vi "Get RTPath String.vi"(8 "error in (no error)":errorcluster, 11 "Target OS in":string) -> (0 "error out":errorcluster, 1 "RT Folder Path":string, 2 "RT File Path":string, 3 "Target OS out":string)   [LabVIEW 2019, in "TLCD System Tests.lvclass"]
uses:
  TLCD System Tests.lvclass
  TLCD Test Class/TLCD Test Class.lvclass
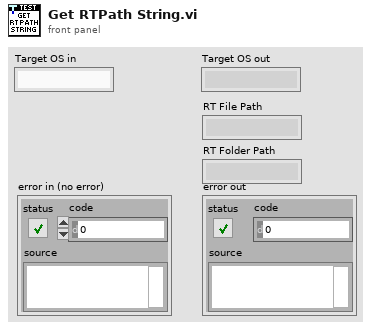
[diagram p1: front panel]
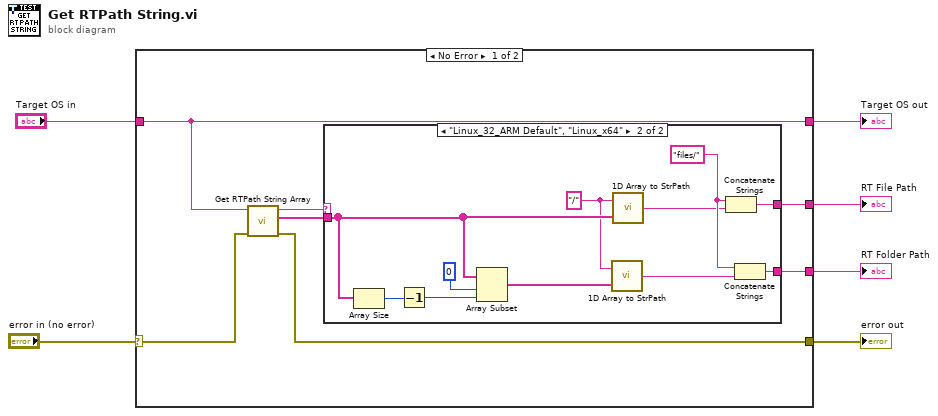
[diagram p0: block diagram]
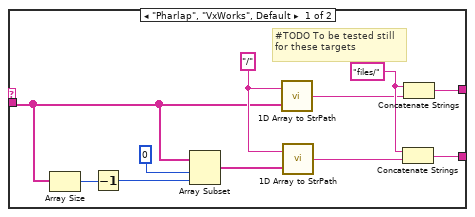
[diagram p2: hidden frame]
diagram:
  n1 = case shown="No Error" "error in (no error)" {
    selector: "error in (no error)" -> [w9 w36]
    tunnel: [w13 _] -> w6
    tunnel: [w12 w36] -> w5
    tunnel: "Target OS in" -> [w8 w37]
    tunnel: [w8 w37] -> w2
    tunnel: [w7 _] -> w1
    frame No Error {
      n2 = call "Get RTPath String Array.vi"("error in (no error)"=w9, "Target OS"=w8) -> ("error out"=w12:errorcluster, "File Path String Array"=w11:string[], "Target OS out"=w10:string)  [unwired: 7 in]
      n3 = case shown="\"Linux_32_ARM Default\", \"Linux_x64\"" w10 {
        tunnel: w11 -> [w16 w31]
        tunnel: [w24 w35] -> w13
        tunnel: [w18 w32] -> w7
        frame "Pharlap", "VxWorks", Default {
          w19 = "files/" ("string")
          w21 = "/" ("delimiter (Tab)")
          # "#TODO To be tested still for these targets"
          n4 = Array Size(array=w16) -> (size(s)=w15:i32)
          n5 = Decrement(x=w15) -> (x-1=w14:i32)
          n6 = Array Subset(array=w16, index=0, length=w14) -> (w22:string[])
          n7 = call "1D Array to StrPath.vi"("File Path String Array"=w16, "Delimiter"=w21) -> ("Path string"=w17:string)
          n8 = call "1D Array to StrPath.vi"("File Path String Array"=w22, "Delimiter"=w21) -> ("Path string"=w20:string)
          n9 = Concatenate Strings(w19, w20) -> (w18:string)
          n10 = Concatenate Strings(w19, w17) -> (w24:string)
        }
        frame "Linux_32_ARM Default", "Linux_x64" {
          w29 = "/" ("Delimiter")
          w33 = "files/" ("string")
          n11 = Array Size(array=w31) -> (size(s)=w26:i32)
          n12 = Decrement(x=w26) -> (x-1=w25:i32)
          n13 = Array Subset(array=w31, index=0, length=w25) -> (w30:string[])
          n14 = call "1D Array to StrPath.vi"("File Path String Array"=w30, "Delimiter"=w29) -> ("Path string"=w27:string)
          n15 = call "1D Array to StrPath.vi"("File Path String Array"=w31, "Delimiter"=w29) -> ("Path string"=w28:string)
          n16 = Concatenate Strings(w33, w28) -> (w35:string)
          n17 = Concatenate Strings(w33, w27) -> (w32:string)
        }
      }
    }
    frame Error {
    }
  }
  "RT File Path" <- w6
  "error out" <- w5
  "Target OS out" <- w2
  "RT Folder Path" <- w1
